vi "get sw timing source name.vi"(11 "sw defined timing source":u8) -> (3 "clock string":string)   [LabVIEW 2013, in "TBM module execution interface.lvclass"]
doc: "R&D does not provide a mechanism for defining a sw timing source by name, only by number (0-127). However, the clock string generated follows a standard format, stored inside of the pw-protected VI. This VI has the same password."
uses:
  TBM module execution interface.lvclass
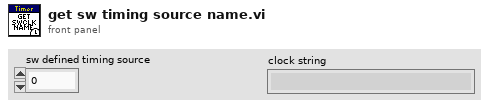
[diagram p1: front panel]
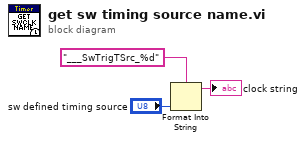
[diagram p0: block diagram]
diagram:
  n1 = Format Into String(format string="___SwTrigTSrc_%d", "sw defined timing source") -> (resulting string=→"clock string":string)  [unwired: 2 in, 1 out]
